vi "Get Constrained Data.vi"(4 "Maximum Magnitude":dbl, 6 "Minimum Magnitude":dbl, 8 "Maximum Angle (DEG)":dbl, 9 "Minimum Angle (DEG)":dbl, 10 "Lidar Directions":dbl[](array[numeric]), 11 "Lidar Magnitudes":dbl[](array[numeric])) -> (2 "Constrained Angles":dbl[](array[numeric]), 3 "Constrained Magnitudes":dbl[](array[numeric]))   [LabVIEW 2016]
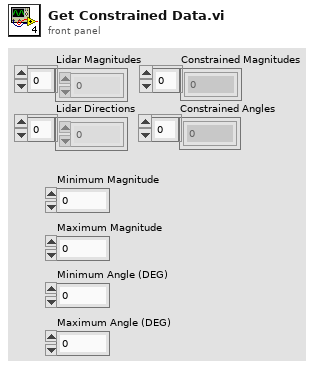
[diagram p1: front panel]
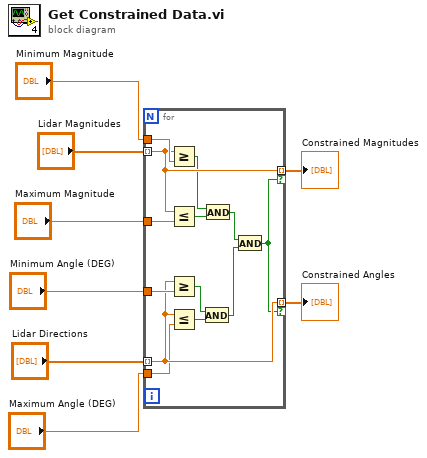
[diagram p0: block diagram]
diagram:
  n1 = for {
    tunnel: [w14] -> w3 mode=indexing if=w11
    tunnel: "Lidar Magnitudes" -> [w14] mode=indexing
    tunnel: [w20] -> w4 mode=indexing if=w11
    tunnel: "Lidar Directions" -> [w20] mode=indexing
    tunnel: "Minimum Angle (DEG)" -> [w21]
    tunnel: "Maximum Angle (DEG)" -> [w19]
    tunnel: "Minimum Magnitude" -> [w16]
    tunnel: "Maximum Magnitude" -> [w15]
    n2 = Greater Or Equal?(x=w14, y=w16) -> (x >= y?=w9:bool)
    n3 = Less Or Equal?(x=w14, y=w15) -> (x <= y?=w10:bool)
    n4 = Greater Or Equal?(x=w20, y=w21) -> (x >= y?=w18:bool)
    n5 = Less Or Equal?(x=w20, y=w19) -> (x <= y?=w17:bool)
    n6 = And(x=w18, y=w17) -> (x .and. y?=w12:bool)
    n7 = And(x=w9, y=w10) -> (x .and. y?=w13:bool)
    n8 = And(x=w13, y=w12) -> (x .and. y?=w11:bool)
  }
  "Constrained Magnitudes" <- w3
  "Constrained Angles" <- w4
